vi "cmd_vi.vi"() -> ()   [LabVIEW 2010]
doc: "Demonstrates how to set up a basic TCP connection, send data to the specified port once a connection has been established, and terminate the connection once the data has been sent. This VI is designed to stop if the TCP connection is terminated.\n\nThe data sent in this example is an array consisting of one of three user selectable waveforms.\n\n<B>Note:</B> Requires the Simple Data Client.vi located in the same library as this VI."
panel:
  out "Out":string
  out "error out":errorcluster
  out "Boolean":bool
  out "data out":string
  in  "stop":bool
  in  "Port":u16=5010 min=1025 step=1
  # "Instructions:\n1. Open the Simple Data Client.vi.\n2. Run this VI first.\n3. Run the Simple Data Client.vi second.\n4. Adjust the Function and # of Points controls to see the plot on the front panel of the Simple Data Client.vi change.\n\nNote:  This VI will time out after 60 seconds if no connection is detected."
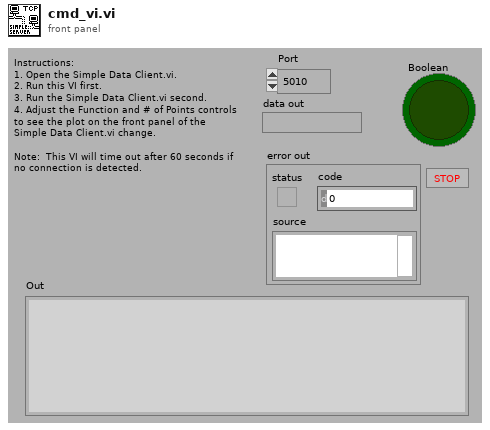
[diagram p1: front panel]
types:
  T1 = enum16{"Standard", "Buffered", "CRLF", "Immediate"}
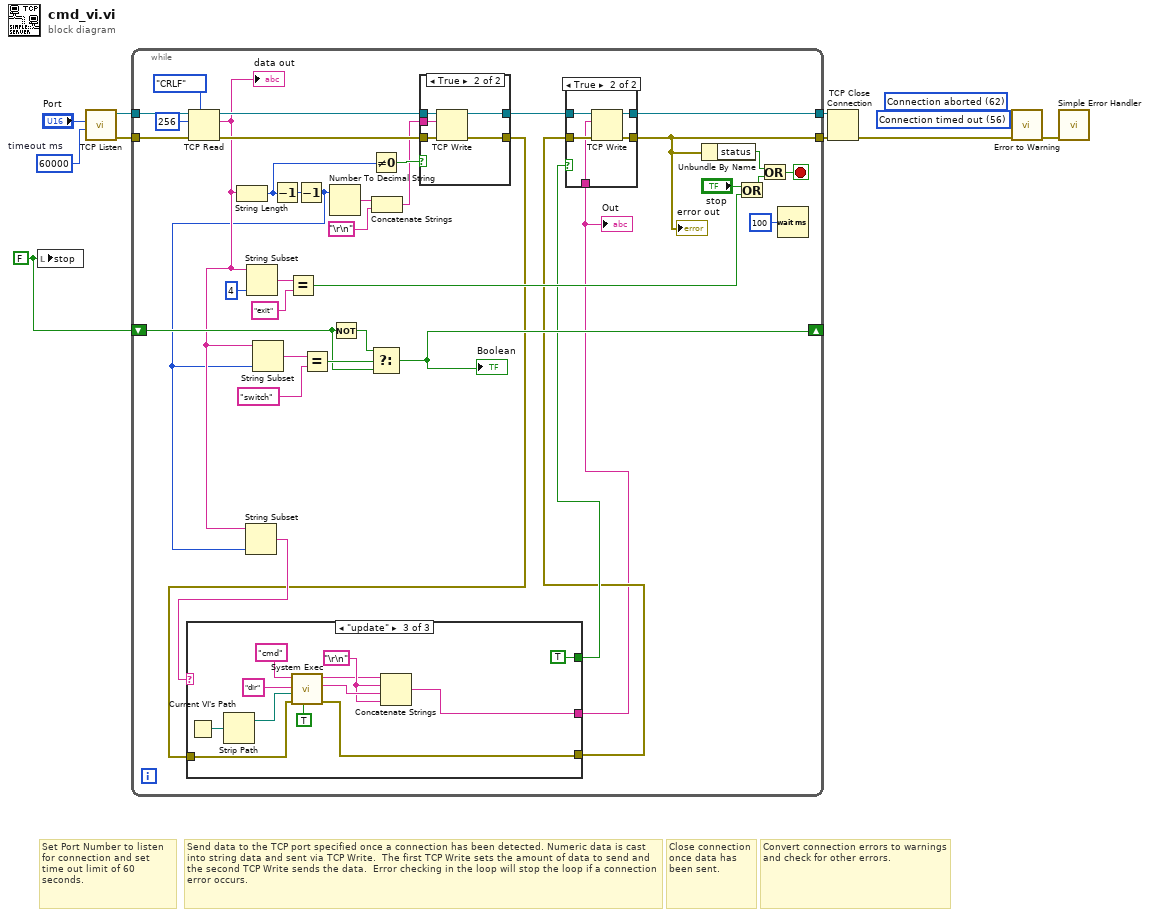
[diagram p0: block diagram]
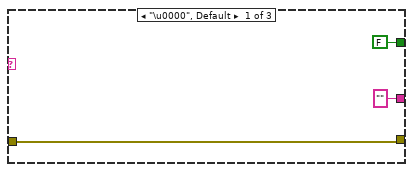
[diagram p2: hidden frame]
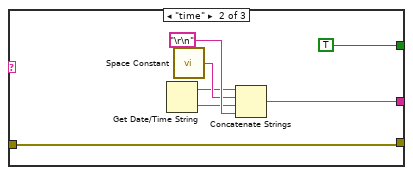
[diagram p3: hidden frame]
diagram:
  w1 = FALSE ("stop")
  w2 = 60000  # timeout ms
  w7 = 56 items=["No Error", "Argument Error", "Memory Full", "Out of Zone", "End of File", "File Already Open", "Generic File IO Error", "File Not Found", "File Permission Error", "Disk Full", "Duplicate Path", "Too Many Files Open", "Not Enabled", "Resource File Not Found", "Cannot Add Resource", "Resource Not Found", "Image Not Found", "Image Memory Error", "Pen Does Not Exist", "Config Bad Type", "Config Token Not Found", "Config Parse Error", "Config Memory Error", "Bad External Code Format", "Bad External Code Offset", "External Code Not Present", "Null Window", "Destroy Window Mixup", "Null Menu", "Print Aborted", "Bad Print Record", "Print Driver Error", "Windows Error During Print", "Memory Error During Print", "Print Dialog Error", "Generic Print Error", "Invalid Device Refnum", "Device Not Found", "Device Parameter Error", "Device Unit Error", "Can't Open Device", "Device Call Aborted", "Generic Error", "Cancelled By User", "Object ID Too Low", "Object ID Too High", "Object Not In Heap", "Unknown Heap", "Bad DefProc ID", "DefProc Not In Table", "Message Out Of Range", "Null Method", "Unknown Message", "Manager Call Not Supported", "Bad address", "Connection In progress", "Connection timed out", "Connection is already in progress", "Network attribute not supported", "Network error", "Address in use", "System out of memory", "Connection aborted", "Connection refused", "Connection is not connected", "Connection is already connected", "Connection closed", "Initialize error (interapplication manager)", "Bad occurrence", "Wait on unbound occurrence handler", "Occurrence queue overflow", "Bad path", "Semaphore not signaled", "Unrecognized type (interapplication manager)"] ("2nd Error to Convert")
  w8 = 62 items=["No Error", "Argument Error", "Memory Full", "Out of Zone", "End of File", "File Already Open", "Generic File IO Error", "File Not Found", "File Permission Error", "Disk Full", "Duplicate Path", "Too Many Files Open", "Not Enabled", "Resource File Not Found", "Cannot Add Resource", "Resource Not Found", "Image Not Found", "Image Memory Error", "Pen Does Not Exist", "Config Bad Type", "Config Token Not Found", "Config Parse Error", "Config Memory Error", "Bad External Code Format", "Bad External Code Offset", "External Code Not Present", "Null Window", "Destroy Window Mixup", "Null Menu", "Print Aborted", "Bad Print Record", "Print Driver Error", "Windows Error During Print", "Memory Error During Print", "Print Dialog Error", "Generic Print Error", "Invalid Device Refnum", "Device Not Found", "Device Parameter Error", "Device Unit Error", "Can't Open Device", "Device Call Aborted", "Generic Error", "Cancelled By User", "Object ID Too Low", "Object ID Too High", "Object Not In Heap", "Unknown Heap", "Bad DefProc ID", "DefProc Not In Table", "Message Out Of Range", "Null Method", "Unknown Message", "Manager Call Not Supported", "Bad address", "Connection In progress", "Connection timed out", "Connection is already in progress", "Network attribute not supported", "Network error", "Address in use", "System out of memory", "Connection aborted", "Connection refused", "Connection is not connected", "Connection is already connected", "Connection closed", "Initialize error (interapplication manager)", "Bad occurrence", "Wait on unbound occurrence handler", "Occurrence queue overflow", "Bad path", "Semaphore not signaled", "Unrecognized type (interapplication manager)"] ("1st Error to Convert")
  # "Convert connection errors to warnings and check for other errors."
  # "Close connection once data has been sent."
  # "Send data to the TCP port specified once a connection has been detected. Numeric data is cast into string data and sent via TCP Write.  The first TCP Write sets the amount of data to send and the second TCP Write sends the data.  Error checking in the loop will stop the loop if a connection error occurs."
  # "Set Port Number to listen for connection and set time out limit of 60 seconds."
  n1 = local write "stop"(w1) -> ()
  n2 = call <vilib>:"TCP Listen.vi"("timeout ms (wait forever: -1)"=w2, "port"="Port") -> ("error out"=w3:errorcluster, "connection ID"=w5:refnum<k5>)  [unwired: 6 in, 2 out]
  n3 = while {
    tunnel: [w19] -> w4
    tunnel: [w20] -> w6
    tunnel: w5 -> [w47]
    tunnel: w3 -> [w43]
    shift-right: [w21] -> _
    shift-left: w1 -> [w22]
    stop <- w45 stop-if-true
    n4 = TCP Read(connection ID=w47, bytes to read=256, 7:T1."CRLF" ("mode (standard)")) -> (connection ID out=w40:refnum<k5>, data out=w18:string)  [unwired: 2 in, 1 out]
    "data out" <- w18
    n5 = String Length(string=w18) -> (length=w37:i32)
    n6 = String Subset(string=w18, length (rest)=4 ("length (rest)")) -> (substring=w33:string)  [unwired: 1 in]
    n7 = Decrement(x=w37) -> (x-1=w28:i32)
    n8 = Equal?(x=w33, y="exit") -> (x = y?=w31:bool)
    n9 = Decrement(x=w28) -> (x-1=w17:i32)
    n10 = String Subset(string=w18, length (rest)=w17) -> (substring=w16:string)  [unwired: 1 in]
    n11 = String Subset(string=w18, length (rest)=w17) -> (substring=w26:string)  [unwired: 1 in]
    n12 = Equal?(x=w26, y="switch" ("search string")) -> (x = y?=w24:bool)
    n13 = Number To Decimal String(number=w17) -> (decimal integer string=w39:string)  [unwired: 1 in]
    n14 = Not(x=w22) -> (.not. x?=w23:bool)
    n15 = Not Equal To 0?(x=w37) -> (x != 0?=w38:bool)
    n16 = Select(t=w23, s=w24, f=w22) -> (s? t:f=w21:bool)
    "Boolean" <- w21
    n17 = Concatenate Strings(w39, "\r\n") -> (w30:string)
    n18 = case shown="True" w38 {
      tunnel: w43 -> [w77 w83]
      tunnel: [w77 w82] -> w14
      tunnel: [w78 w81] -> w41
      tunnel: w40 -> [w78 w80]
      tunnel: w30 -> [_ w79]
      frame False {
      }
      frame True {
        n19 = TCP Write(connection ID=w80, data in=w79, error in (no error)=w83) -> (connection ID out=w81:refnum<k5>, error out=w82:errorcluster)  [unwired: 1 in, 1 out]
      }
    }
    n20 = case shown="\"update\"" w16 {
      tunnel: [FALSE TRUE TRUE] -> w15
      tunnel: ["" w52 w58] -> w12
      tunnel: [w48 w51 w64] -> w13
      tunnel: w14 -> [w48 w51 w63]
      frame "\u0000", Default {
      }
      frame "time" {
        n21 = Get Date/Time String() -> (date string=w54:string, time string=w56:string)  [unwired: 3 in]
        n22 = call <vilib>:"Space Constant.vi"() -> ("String"=w55:string)
        n23 = Concatenate Strings(w54, w55, w56, "\r\n") -> (w52:string)
      }
      frame "update" {
        w65 = "\r\n"
        n24 = Current VI's Path() -> (path=w61:path)
        n25 = Strip Path(path=w61) -> (stripped path=w60:path)  [unwired: 1 out]
        n26 = call <vilib>:"System Exec.vi"("run minimized? (F)"=TRUE, "error in (no error)"=w63, "working directory"=w60, "standard input"="dir" ("command line"), "command line"="cmd") -> ("error out"=w64:errorcluster, "standard error"=w66:string, "standard output"=w59:string)  [unwired: 3 in, 1 out]
        n27 = Concatenate Strings(w59, w65, w66, w65) -> (w58:string)
      }
    }
    "Out" <- w12
    n28 = case shown="True" w15 {
      tunnel: w41 -> [w71 w76]
      tunnel: [w71 w75] -> w20
      tunnel: w13 -> [w70 w74]
      tunnel: [w70 w73] -> w19
      tunnel: w12 -> [_ w72]
      frame False {
      }
      frame True {
        n29 = TCP Write(connection ID=w76, data in=w72, error in (no error)=w74) -> (connection ID out=w75:refnum<k5>, error out=w73:errorcluster)  [unwired: 1 in, 1 out]
      }
    }
    "error out" <- w19
    n30 = Unbundle By Name(w19) -> ("status"=w44:bool)
    n31 = Or(x="stop", y=w31) -> (x .or. y?=w32:bool)
    n32 = Or(x=w44, y=w32) -> (x .or. y?=w45:bool)
    n33 = Wait (ms)(milliseconds to wait=u32 100) -> ()  [unwired: 1 out]
  }
  n34 = TCP Close Connection(connection ID=w6, error in (no error)=w4) -> (error out=w10:errorcluster)  [unwired: 1 in, 1 out]
  n35 = call <vilib>:"Error to Warning.vi"("1st Error to Convert"=w8, "2nd Error to Convert"=w7, "error in"=w10) -> ("warning out"=w9:errorcluster)  [unwired: 12 in]
  n36 = call <vilib>:"Simple Error Handler.vi"("error in (no error)"=w9) -> ()  [unwired: 4 in, 5 out]
